vi "Write Use System Alert_.vi"(8 "error in (no error)":errorcluster, 10 "Use System Alert?":bool, 11 "Write Beep Parameters Msg in":refnum<class "Write Beep Parameters Msg.lvclass">) -> (0 "error out":errorcluster, 3 "Write Beep Parameters Msg out":refnum<class "Write Beep Parameters Msg.lvclass">)   [LabVIEW 2016, in "CS++BeepActor.lvlib" / "Write Beep Parameters Msg.lvclass"]
uses:
  Write Beep Parameters Msg.lvclass
  Write Beep Parameters Msg.lvclass/Write Beep Parameters Msg.ctl
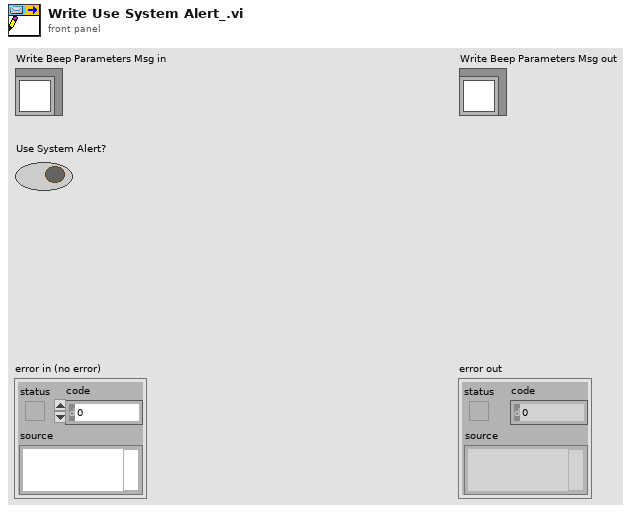
[diagram p1: front panel]
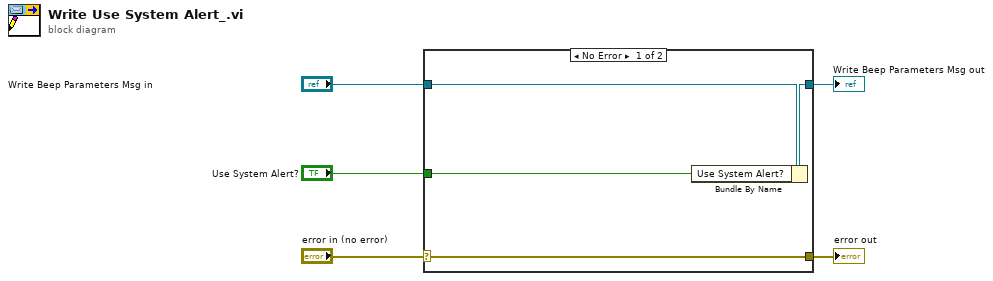
[diagram p0: block diagram]
diagram:
  n1 = case shown="No Error" "error in (no error)" {
    selector: "error in (no error)" -> [w9 w10]
    tunnel: [w9 w10] -> w4
    tunnel: [w7 w11] -> w2
    tunnel: "Write Beep Parameters Msg in" -> [w8 w11]
    tunnel: "Use System Alert?" -> [w6 _]
    frame No Error {
      n2 = Bundle By Name(cluster=w8, "Use System Alert?"=w6) -> (w7:refnum<class "Write Beep Parameters Msg.lvclass">)
    }
    frame Error {
    }
  }
  "error out" <- w4
  "Write Beep Parameters Msg out" <- w2
